vi "Coriolis Torque.vi"   [LabVIEW 2017, in "NI_Kinematics.lvlib"]
doc: "Calculates the joint torques that result from the Coriolis and centripetal forces on the joints of a robotic arm. Wire data to the <B>joint positions</B> input to determine the polymorphic instance to use or manually select the instance. \n\n<B>.m file:</B> coriolis"
uses:
  <vilib>/robotics/Kinematics/NI_Kinematics.lvlib
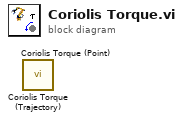
[diagram p0: block diagram]
diagram:
  n1 = call <vilib>:"Coriolis Torque (Trajectory).vi"() -> ()  [unwired: 9 in, 3 out]
  n2 = call <vilib>:"Coriolis Torque (Point).vi"() -> ()  [unwired: 9 in, 3 out]
